vi "UI_simpleError.vi"(7 "command":string, 8 "error in (no error)":errorcluster, 11 "error stop":refnum<user-event>) -> (0 "error out":errorcluster)   [LabVIEW 2020]
panel:
  out "source":string
  out "code":i32
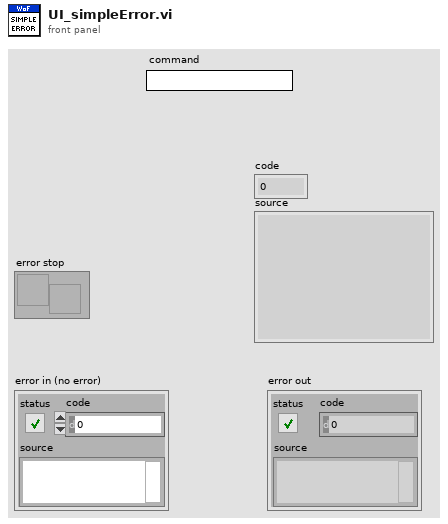
[diagram p1: front panel]
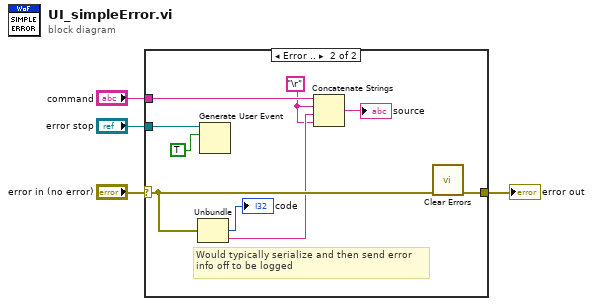
[diagram p0: block diagram]
diagram:
  n1 = case shown="Error .." "error in (no error)" {
    selector: "error in (no error)" -> [w5 w11]
    tunnel: "error stop" -> [_ w14]
    tunnel: [w5 w12] -> w2
    tunnel: "command" -> [_ w9]
    frame No Error {
    }
    frame Error {
      w7 = "\r"
      # "Would typically serialize and then send error\ninfo off to be logged"
      n2 = Unbundle(w11) -> ("code"=→"code":i32, "source"=w8:string)  [unwired: 1 out]
      n3 = Generate User Event(user event=w14, event data cluster=TRUE ("event data")) -> ()  [unwired: 2 in, 2 out]
      n4 = Concatenate Strings(w9, w7, w8, w7) -> (→"source":string)
      n5 = call <vilib>:"Clear Errors.vi"("error in (no error)"=w11) -> ("error out"=w12:errorcluster)  [unwired: 5 in, 1 out]
    }
  }
  "error out" <- w2
